vi "Get Fastest Recommended VS Speed.vi"(8 "error in (no error)":errorcluster, 10 "speed":sgl, 11 "index":i32) -> (0 "error out":errorcluster, 1 "function return":u32, 2 "speed out":sgl, 3 "index out":i32)   [LabVIEW 2014, in "atmcd32d.lvlib"]
doc: "unsigned int WINAPI GetFastestRecommendedVSSpeed(int * index, float * speed);"
uses:
  atmcd32d.lvlib
  atmcd32d.dll
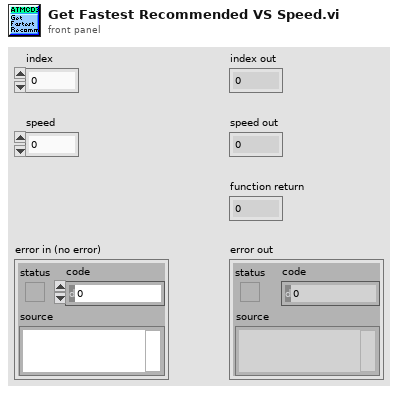
[diagram p1: front panel]
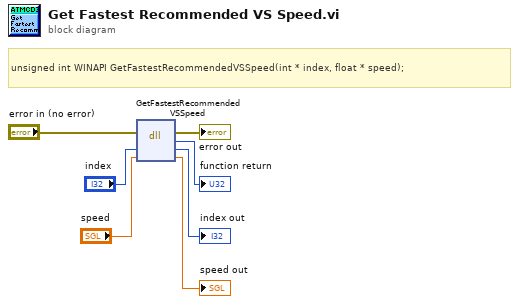
[diagram p0: block diagram]
diagram:
  # "unsigned int WINAPI GetFastestRecommendedVSSpeed(int * index, float * speed);"
  n1 = dll-call lib="C:/Users/Bakir/Documents/Lambda2-Testing/lib/Andorlib/atmcd32d.*" fn="GetFastestRecommendedVSSpeed"(error in="error in (no error)", "index"="index", "speed"="speed") -> (error out=→"error out":errorcluster, →"function return":u32, "index"=→"index out":i32, "speed"=→"speed out":sgl)  [unwired: 2 in, 1 out]
